vi "2_04.vi"   [LabVIEW 2018]
uses:
  <vilib>/Analysis/3filter.llb/Chebyshev Filter (DBL).vi
  <vilib>/Analysis/NI_AALBase.lvlib
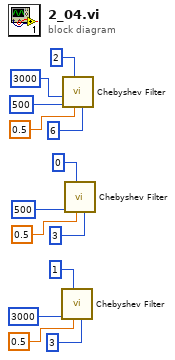
[diagram p0: block diagram]
diagram:
  n1 = call-poly <vilib>:"Chebyshev Filter.vi"("order"=3, "ripple(dB)"=0.5, "filter type"=1, "low cutoff freq: fl"=3000) -> ()  [unwired: 6 in, 2 out]
  n2 = call-poly <vilib>:"Chebyshev Filter.vi"("order"=6, "ripple(dB)"=0.5, "filter type"=2, "low cutoff freq: fl"=500, "high cutoff freq: fh"=3000) -> ()  [unwired: 5 in, 2 out]
  n3 = call-poly <vilib>:"Chebyshev Filter.vi"("order"=3, "ripple(dB)"=0.5, "filter type"=0, "low cutoff freq: fl"=500) -> ()  [unwired: 6 in, 2 out]
